vi "Write State.vi"(8 "error in (no error)":errorcluster, 10 "state":T1, 11 "Framework in":refnum<class "Framework.lvclass">) -> (0 "error out":errorcluster, 3 "Framework out":refnum<class "Framework.lvclass">)   [LabVIEW 2020, in "DSF Core.lvlib" / "Framework.lvclass"]
uses:
  Framework.lvclass
  <vilib>/NI/Memory Manager/Classes/Pointer/Pointer.lvclass
  <vilib>/NI/Memory Manager/Classes/Pointer/Write U8.vi
  Framework States.ctl
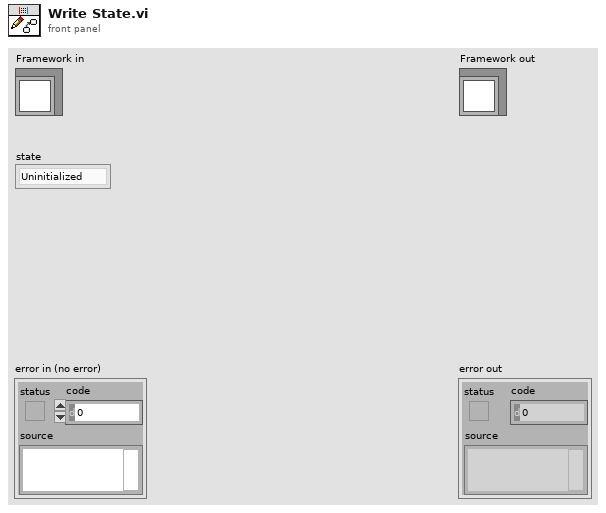
[diagram p1: front panel]
types:
  T1 = typedef "DSF Core.lvlib/Framework.lvclass/Framework States.ctl" = enum8{"Uninitialized", "Initialized", "Start", "Rx", "Tx", "Shutdown"}
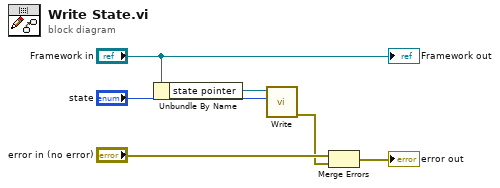
[diagram p0: block diagram]
diagram:
  n1 = Unbundle By Name("Framework in") -> ("state pointer"=w5:refnum<class "Pointer.lvclass">)
  n2 = call-poly <vilib>:"Write.vi"("value"="state", "Pointer in"=w5) -> ("error out"=w1:errorcluster)  [unwired: 6 in, 3 out]
  n3 = Merge Errors("error in (no error)", w1) -> (→"error out":errorcluster)
  "Framework out" <- "Framework in"
